vi "TempCtl_test.vi"(2 "shiftReg":bool, 3 "enable":bool, 4 "Hysterese":sgl, 5 "Soll":sgl, 6 "IST":dbl, 7 "heating":bool) -> (0 "shiftReg":bool, 1 "heating":bool)   [LabVIEW 2011]
panel:
  in  "stop":bool
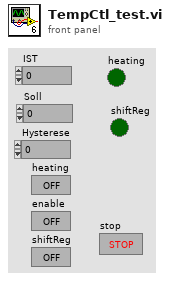
[diagram p1: front panel]
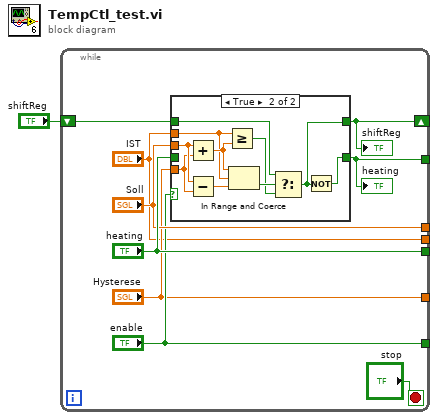
[diagram p0: block diagram]
diagram:
  n1 = while {
    tunnel: ["IST"] -> _
    tunnel: ["enable"] -> _
    tunnel: ["heating"] -> _
    tunnel: ["Hysterese"] -> _
    tunnel: ["Soll"] -> _
    tunnel: [w8] -> _
    shift-right: [w7] -> _
    shift-left: "shiftReg" -> [w10]
    stop <- "stop" stop-if-true
    n2 = case shown="True" "enable" {
      tunnel: "Soll" -> [_ w18]
      tunnel: "Hysterese" -> [_ w17]
      tunnel: [w12 w16] -> w8
      tunnel: "heating" -> [w12 _]
      tunnel: "IST" -> [_ w15]
      tunnel: w10 -> [w11 w14]
      tunnel: [w11 w13] -> w7
      frame False {
      }
      frame True {
        n3 = Add(x=w18, y=w17) -> (x+y=w20:sgl)
        n4 = Subtract(x=w18, y=w17) -> (x-y=w22:sgl)
        n5 = Greater Or Equal?(x=w15, y=w20) -> (x >= y?=w19:bool)
        n6 = In Range and Coerce(upper limit=w20, x=w15, lower limit=w22) -> (In Range?=w21:bool)  [unwired: 1 out]
        n7 = Select(t=w14, s=w21, f=w19) -> (s? t:f=w13:bool)
        n8 = Not(x=w13) -> (.not. x?=w16:bool)
      }
    }
    "heating" <- w8
    "shiftReg" <- w7
  }
